vi "Configure Protocol Settings.vi"(8 "error in":errorcluster, 11 "Protocol settings":T1={"Protocol capture resource name"="", "Clock rate"=12288000, "Number of words"=19200, "Sensitivity"=0.34762, "Protocol"=""}) -> (0 "error out":errorcluster, 3 "PDM task":T2)   [LabVIEW 2021]
uses:
  <vilib>/PDM Acquisition Toolkit/host/Classes/Tasks/PCM Input/Controls/DVR PCM Input Task.ctl
  <vilib>/PDM Acquisition Toolkit/host/Classes/Tasks/PCM Input/PCM Input Task.lvclass
  controls/Protocol settings.ctl
  <vilib>/PDM Acquisition Toolkit/host/Classes/Tasks/PDM Tasks/Controls/Acquisition Mode.ctl
  <vilib>/PDM Acquisition Toolkit/host/Classes/Session/Controls/Logic Levels.ctl
  <vilib>/PDM Acquisition Toolkit/shared/controls/PCM Data Format Configuration.ctl
  <vilib>/PDM Acquisition Toolkit/shared/controls/Digital Edge.ctl
  <vilib>/PDM Acquisition Toolkit/shared/controls/PCM Bit Endianness.ctl
  <vilib>/PDM Acquisition Toolkit/shared/controls/PCM Data Justification.ctl
  <vilib>/PDM Acquisition Toolkit/shared/controls/PCM Frame Sync Control.ctl
  <vilib>/PDM Acquisition Toolkit/host/API/Public/Create Tasks/Create PCM Input Task.vi
  <vilib>/PDM Acquisition Toolkit/host/API/Public/Configure/Timing/Configure Timing - PCM Input Slave.vi
  <vilib>/PDM Acquisition Toolkit/host/API/Public/Configure/PDM Channel/Configure Microphone Sensitivity FSPA - PCM Input Task.vi
  <vilib>/PDM Acquisition Toolkit/host/Classes/Tasks/PDM Tasks/PDM Task.lvclass
  <vilib>/PDM Acquisition Toolkit/host/Classes/Session/DecoderSession.lvclass
  <vilib>/PDM Acquisition Toolkit/host/API/PDM Acquisition Toolkit.lvlib
  <vilib>/PDM Acquisition Toolkit/shared/PDM Shared.lvlib
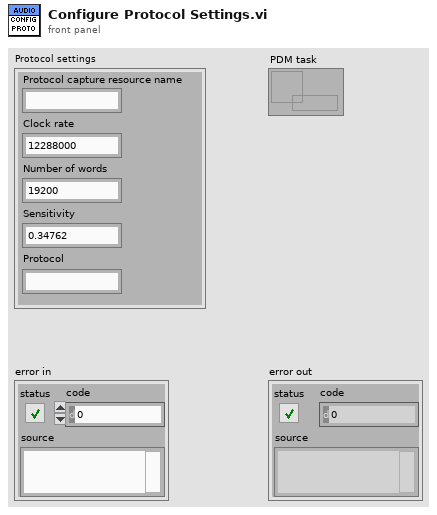
[diagram p1: front panel]
types:
  T1 = typedef "Protocol settings.ctl" = cluster{"Protocol capture resource name":string, "Clock rate":u32, "Number of words":i32, "Sensitivity":dbl, "Protocol":string}
  T2 = typedef "PDM Acquisition Class Library.lvlib/PCM Input Task.lvclass/DVR PCM Input Task.ctl" = refnum<data-value>
  T3 = typedef "PDM Shared.lvlib/PCM Frame Sync Control.ctl" = cluster{"Frame Length":u16, "Frame Sync Pulse Width":u16, "Bit Clock Edge  Sync":T4}
  T4 = typedef "PDM Shared.lvlib/Digital Edge.ctl" = enum8{"Rising", "Falling"}
  T5 = typedef "PDM Shared.lvlib/PCM Data Format Configuration.ctl" = cluster{"Frame Sync Edge for Channel 0":T4, "Channel Count Per Frame":u8, "Channel Length":u16, "Bit Depth":u8, "Channel 0 Offset":u16, "Endianness":T6, "Data Justification":T7}
  T6 = typedef "PDM Shared.lvlib/PCM Bit Endianness.ctl" = enum16{"MSB First", "LSB First"}
  T7 = typedef "PDM Shared.lvlib/PCM Data Justification.ctl" = enum16{"Left Justified", "Right Justified"}
  T8 = typedef "PDM Acquisition Class Library.lvlib/DecoderSession.lvclass/Logic Levels.ctl" = enum16{"3.3 V", "1.8 V", "1.2 V"}
  T9 = typedef "PDM Acquisition Class Library.lvlib/PDM Task.lvclass/Acquisition Mode.ctl" = enum16{"Finite", "Continuous"}
  T10 = cluster{"Frame_Sync_Edge_for_Channel 0":i32, "Channel_Count_Per_Frame":i32, "Channel_Length":i32, "Bit_Depth":i32, "Channel_0_Offset":i32, "Endianness":i32, "Data_Justification":i32, "Frame_Length":i32, "Frame_Sync_Pulse_Width":i32, "Bit_Clock_Edge_Sync":i32}
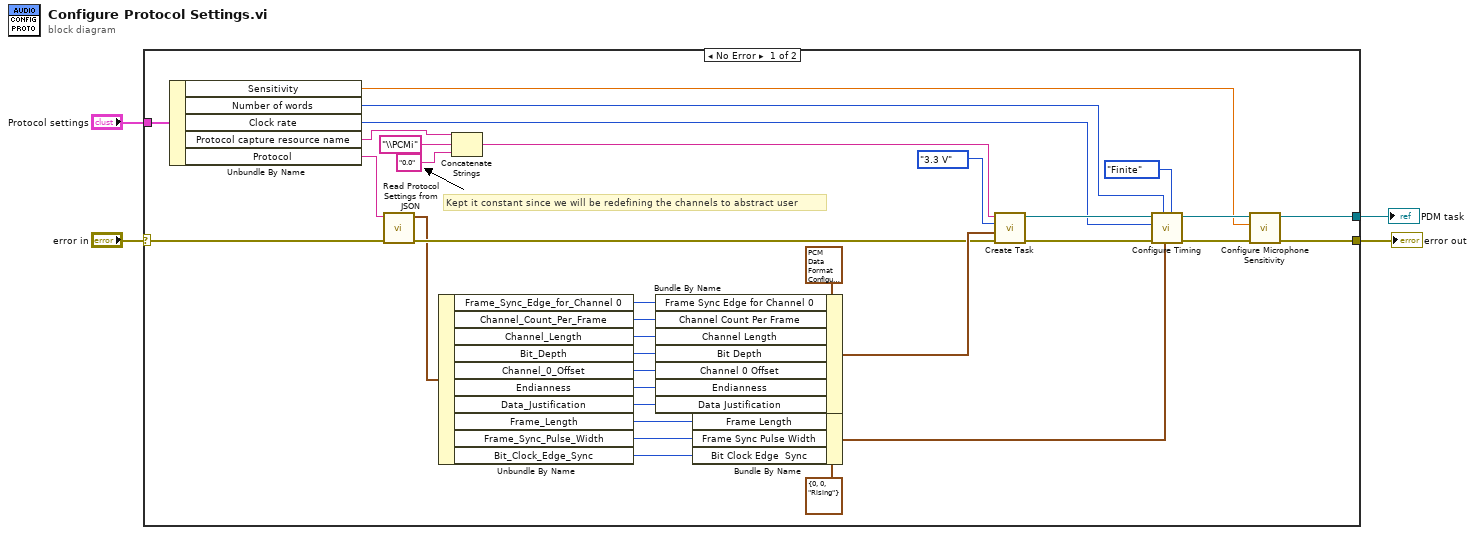
[diagram p0: block diagram]
diagram:
  n1 = case shown="No Error" "error in" {
    selector: "error in" -> [w23 w39]
    tunnel: [w30 w39] -> w2
    tunnel: [w31 _] -> w3
    tunnel: "Protocol settings" -> [w24 _]
    frame No Error {
      # "Kept it constant since we will be redefining the channels to abstract user"
      n2 = Unbundle By Name(w24) -> ("Sensitivity"=w27:dbl, "Number of words"=w26:i32, "Clock rate"=w25:u32, "Protocol capture resource name"=w34:string, "Protocol"=w6:string)
      n3 = call "Read Protocol Settings from JSON.vi"("error in"=w23, "JSON file"=w6) -> ("error out"=w18:errorcluster, "Configurations"=w7:T10)  [unwired: 8 in]
      n4 = Unbundle By Name(w7) -> ("Frame_Sync_Edge_for_Channel 0"=w17:i32, "Channel_Count_Per_Frame"=w16:i32, "Channel_Length"=w15:i32, "Bit_Depth"=w14:i32, "Channel_0_Offset"=w13:i32, "Endianness"=w12:i32, "Data_Justification"=w11:i32, "Frame_Length"=w9:i32, "Frame_Sync_Pulse_Width"=w10:i32, "Bit_Clock_Edge_Sync"=w8:i32)
      n5 = Concatenate Strings(w34, "\\PCMi" ("element"), "0.0" ("string")) -> (w32:string)
      n6 = Bundle By Name(cluster=T5 {"Frame Sync Edge for Channel 0"=enum."Rising", "Channel Count Per Frame"=0, "Channel Length"=0, "Bit Depth"=0, "Channel 0 Offset"=0, "Endianness"=enum."MSB First", "Data Justification"=enum."Left Justified"} ("PCM Data Configuration"), "Frame Sync Edge for Channel 0"=w17, "Channel Count Per Frame"=w16, "Channel Length"=w15, "Bit Depth"=w14, "Channel 0 Offset"=w13, "Endianness"=w12, "Data Justification"=w11) -> (w21:T5)
      n7 = Bundle By Name(cluster=T3 {"Frame Length"=0, "Frame Sync Pulse Width"=0, "Bit Clock Edge  Sync"=enum."Rising"} ("Frame Sync Control"), "Frame Length"=w9, "Frame Sync Pulse Width"=w10, "Bit Clock Edge  Sync"=w8) -> (w19:T3)
      n8 = call-poly <vilib>:"Create Task.vi"("error in"=w18, "PCM data configuration"=w21, "logic level"=Logic_Levels."3.3 V", "channel list"=w32) -> ("error out"=w37:errorcluster, "PCM input task out"=w38:T2)  [unwired: 6 in]
      n9 = call-poly <vilib>:"Configure Timing.vi"("acquisition mode"=Acquisition_Mode."Finite", "Frame Sync Clock Control"=w19, "number of words per channel"=w26, "error in"=w37, "Bit Clock rate"=w25, "PCM input task in"=w38) -> ("error out"=w28:errorcluster, "PCM input task out"=w29:T2)  [unwired: 4 in]
      n10 = call-poly <vilib>:"Configure Microphone Sensitivity.vi"("error in"=w28, "microphone sensitivity (FS/Pa)"=w27, "PCM input task in"=w29) -> ("error out"=w30:errorcluster, "PCM input task out"=w31:T2)  [unwired: 7 in]
    }
    frame Error {
    }
  }
  "PDM task" <- w3
  "error out" <- w2
